vi "HistogramPlot.vi"(4 "Zen Analytics in":refnum<class "Zen Analytics.lvclass">, 6 "Reduced 2D":dbl[][](array[numeric]), 7 "Initialization input":dbl[][](array[numeric]), 8 "error in (no error)":errorcluster, 9 "Graph Refference's":T2, 10 "IndexOfMeasurement":i32, 11 "Plot Cluster":T1) -> (0 "error out":errorcluster, 5 "InitializationOutput":dbl[][](array[numeric]))   [LabVIEW 2019, in "Zen Analytics.lvlib" / "Zen Analytics.lvclass"]
uses:
  Zen Analytics.lvclass
  Dependency/GraphReff.ctl
  Dependency/Plot Cluster.ctl
types:
  T1 = typedef "Zen Analytics.lvlib/Zen Analytics.lvclass/Plot Cluster.ctl" = cluster{"Reduced 2D":dbl[][], "Start Index":i32, "No Of New Termnals":i32, "Top/Bottom":bool, "Values Inserted":i32, "Re-Initialised":bool, "Statistical params":string[][], "MeasurementInitializationData":cluster{"Measurement-ID":i32[], "Measurement Names":string[], "NominalValues":dbl[], "LSL":dbl[], "USL":dbl[], "LCL":dbl[], "UCL":dbl[]}, "MeasurementData":cluster{"Measurement ID":i32, "Measurement Name":string, "Nominal Values":dbl, "LSL":dbl, "USL":dbl, "LCL":dbl, "UCL":dbl}[], "ResultData2D":dbl[][], "PlotParameters":cluster{"Trend":cluster{"TrendPlotID":dbl, "PlotProperties":cluster{"FontName":string, "FontSize":dbl, "FontColor":string, "IsBold":bool, "IsItalic":bool, "PlotColor":string}}[], "Histogram":cluster{"HistogramPlotID":dbl, "PlotProperties":cluster{"FontName":string, "FontSize":dbl, "FontColor":string, "IsBold":bool, "IsItalic":bool, "PlotColor":string}}[], "BarPlot":cluster{"BarPlotID":dbl, "BarValuesID":dbl, "PlotProperties":cluster{"FontName":string, "FontSize":dbl, "IsBold":bool, "IsItalic":bool, "FontColor":string}, "Sectors":string[]}[], "PieChart":cluster{"PieChartID":dbl, "PieChartValueID":dbl, "PlotProperties":cluster{"FontName":string, "FontSize":dbl, "IsBold":bool, "IsItalic":bool, "FontColor":string}, "Sectors":string[]}[]}}
  T2 = typedef "Zen Analytics.lvlib/Zen Analytics.lvclass/GraphReff.ctl" = cluster{"HistgramGraph-reff":refnum<vi>[], "BarGraph-reff":refnum<vi>[], "PieGraph-reff":refnum<vi>[], "Lable-reff":refnum<vi>[], "TrendGraph-reff":refnum<vi>[], "CpCpkTable":refnum<vi>}
  T3 = cluster{"Measurement-ID":i32[], "Measurement Names":string[], "NominalValues":dbl[], "LSL":dbl[], "USL":dbl[], "LCL":dbl[], "UCL":dbl[]}
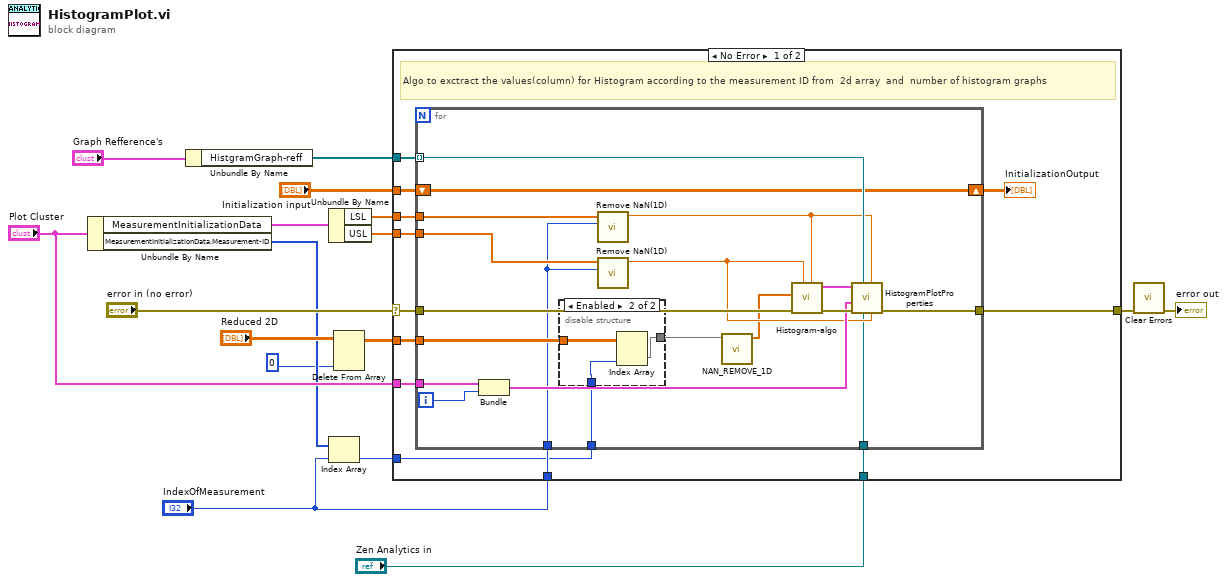
[diagram p0: block diagram]
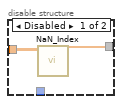
[diagram p2: hidden frame]
diagram:
  n1 = Unbundle By Name("Plot Cluster") -> ("MeasurementInitializationData"=w8:T3, "MeasurementInitializationData.Measurement-ID"=w6:i32[])
  n2 = Unbundle By Name("Graph Refference's") -> ("HistgramGraph-reff"=w14:refnum<vi>[])
  n3 = Unbundle By Name(w8) -> ("LSL"=w13:dbl[], "USL"=w12:dbl[])
  n4 = Index Array(array=w6, index="IndexOfMeasurement") -> (element=w4:i32)
  n5 = Delete From Array(array="Reduced 2D", index (col)=0 ("index")) -> (array with subset deleted=w3:dbl[][])  [unwired: 2 in, 1 out]
  n6 = case shown="No Error" "error in (no error)" {
    selector: "error in (no error)" -> [w24 w54]
    tunnel: [w23 w54] -> w16
    tunnel: w13 -> [w29 _]
    tunnel: w12 -> [w28 _]
    tunnel: w14 -> [w26 _]
    tunnel: w3 -> [w27 _]
    tunnel: "Plot Cluster" -> [w25 _]
    tunnel: "Initialization input" -> [w22 _]
    tunnel: "IndexOfMeasurement" -> [w20 _]
    tunnel: w4 -> [w19 _]
    tunnel: "Zen Analytics in" -> [w18 _]
    frame No Error {
      # "Algo to exctract the values(column) for Histogram according to the measurement ID from  2d array  and  number of histogram graphs"
      n7 = for {
        tunnel: [w41] -> w23
        tunnel: w24 -> [w42]
        tunnel: w29 -> [w39]
        tunnel: w28 -> [w37]
        tunnel: w27 -> [w40]
        tunnel: w26 -> [w47] mode=indexing
        tunnel: w25 -> [w44]
        tunnel: w20 -> [w35]
        shift-right: [w34] -> w21
        shift-left: w22 -> [w34]
        tunnel: w19 -> [w33]
        tunnel: w18 -> [w32]
        i -> [w45]
        n8 = Bundle("Plot Cluster"=w44, w45) -> (w43:cluster{"Plot Cluster":T1, i32})  [unwired: 1 in]
        n9 = disable-structure shown="Enabled" {
          disable-tunnel: w40 -> [w50 w53]
          disable-tunnel: [w49 w51] -> w31
          disable-tunnel: w33 -> [_ w52]
          frame Disabled {
            n10 = call "NaN_Index.vi"("Input"=w50) -> ("Output"=w49:dbl[])  [unwired: 9 in, 1 out]
          }
          frame Enabled {
            n11 = Index Array(array=w53, index (col)=w52) -> (element=w51:dbl[])  [unwired: 1 in]
          }
        }
        n12 = call "Remove NaN(1D).vi"("Index"=w35, "Input"=w39) -> ("Numeric"=w38:dbl)  [unwired: 9 in]
        n13 = call "Remove NaN(1D).vi"("Index"=w35, "Input"=w37) -> ("Numeric"=w36:dbl)  [unwired: 9 in]
        n14 = call "NAN_REMOVE_1D.vi"("Array 2"=w31) -> ("Array"=w30:dbl[])  [unwired: 10 in]
        n15 = call "Histogram-algo.vi"("LSL"=w38, "USL"=w36, "error in"=w42, "Data"=w30) -> ("error out"=w48:errorcluster, "Histogram Graph"=w46:cluster{dbl[], dbl[]}[])  [unwired: 6 in]
        n16 = call "HistogramPlotProperties.vi"("UCL"=w36, "LCL"=w38, "Zen Analytics in"=w32, "Histogram Summary"=w47, "error in (no error)"=w48, "Plot Cluster Index out"=w43, "HistogramValue"=w46) -> ("error out"=w41:errorcluster)  [unwired: 4 in]
      }
      "InitializationOutput" <- w21
    }
    frame Error {
    }
  }
  n17 = call <vilib>:"Clear Errors.vi"("error in (no error)"=w16) -> ("error out"=→"error out":errorcluster)  [unwired: 5 in, 1 out]
